vi "Update.vi"(7 "Row":i32, 8 "error in (no error)":errorcluster, 9 "Workspace":T1, 10 "Routine":T2=enum."Dispense on Plate", 11 "Assembly Run in":refnum<class "Assembly Run.lvclass">) -> (0 "error out":errorcluster, 3 "Assembly Run out":refnum<class "Assembly Run.lvclass">)   [LabVIEW 2021, in "Assembly Run.lvclass"]
uses:
  Assembly Run.lvclass
  Routine/Routine Enum.ctl
  Workspace/Fixture Enum.ctl
  Assembly Run.lvclass/Assembly Run.ctl
  Routine/Routine.lvclass
  Workspace/Fixture.lvclass
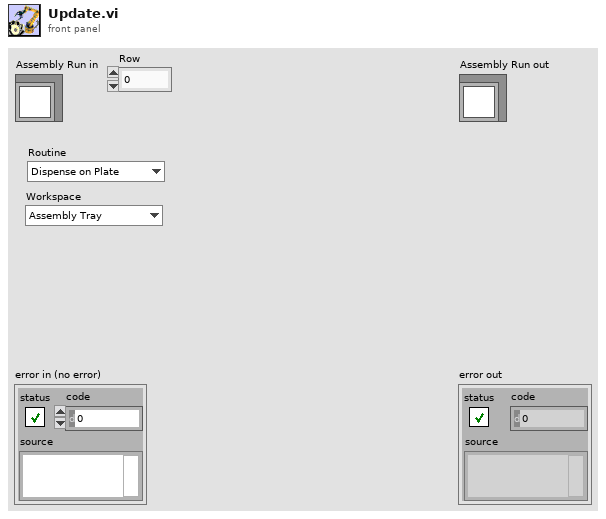
[diagram p1: front panel]
types:
  T1 = typedef "Fixture.lvclass/Fixture Enum.ctl" = enum16{"Assembly Tray", "Syringe Space", "Component", "Pick Up Tool", "Current Position"}
  T2 = typedef "Routine.lvclass/Routine Enum.ctl" = enum16{"Primary Pick Up", "Secondary Pick Up", "Put Down All", "Secure Syringe", "Release Syringe", "Dispense on Plate", "Dispense on Sensor", "Pick Up All", "Put Down Secondary", "Dispense on Kapton"}
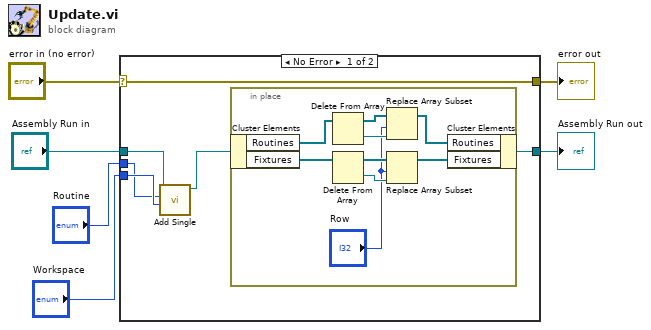
[diagram p0: block diagram]
diagram:
  n1 = case shown="No Error" "error in (no error)" {
    selector: "error in (no error)" -> [w12 w23]
    tunnel: [w12 w23] -> w5
    tunnel: [w11 w22] -> w3
    tunnel: "Assembly Run in" -> [w9 w22]
    tunnel: "Routine" -> [w7 _]
    tunnel: "Workspace" -> [w10 _]
    frame No Error {
      n2 = call-dynamic "Add Single.vi"("Fixture"=w10, "Routine"=w7, "UI in"=w9) -> ("UI out"=w8:refnum<class "Assembly Run.lvclass">)  [unwired: 6 in, 1 out]
      n3 = in-place {
        n4 = in-place-cluster #1(w8) -> ("Routines"=w17:refnum<class "Routine.lvclass">[], "Fixtures"=w16:refnum<class "Fixture.lvclass">[])
        n5 = Delete From Array(array=w17) -> (deleted portion=w19:refnum<class "Routine.lvclass">, array with subset deleted=w18:refnum<class "Routine.lvclass">[])  [unwired: 2 in]
        n6 = Delete From Array(array=w16) -> (deleted portion=w20:refnum<class "Fixture.lvclass">, array with subset deleted=w21:refnum<class "Fixture.lvclass">[])  [unwired: 2 in]
        n7 = Replace Array Subset(array=w18, new element=w19, index="Row") -> (w15:refnum<class "Routine.lvclass">[])
        n8 = Replace Array Subset(array=w21, new element=w20, index="Row") -> (w14:refnum<class "Fixture.lvclass">[])
        n9 = in-place-cluster #1("Routines"=w15, "Fixtures"=w14) -> (w11:refnum<class "Assembly Run.lvclass">)
      }
    }
    frame Error {
    }
  }
  "error out" <- w5
  "Assembly Run out" <- w3
